vi "gripper.vi"() -> ()   [LabVIEW 2017]
uses:
  Program Files (x86)/National Instruments/LabVIEW 2017/examples/Instrument IO/Serial/support/Serial - Settings.ctl
  <vilib>/Instr/_visa.llb/VISA Configure Serial Port (Instr).vi
panel:
  in  "열림":bool
  in  "닫힘":bool
  out "입력":string="*IDN?\n"
  in  "정지":bool
  out "Response":string
  out "bytes read":u32
  out "check":bool
  in  "Serial Settings":T1={"baud rate"=9600, "data bits"=8, "parity"=enum."None", "stop bits"=10, "flow control"=0} {"flow control" items=["None"=0, "XON/XOFF"=1, "RTS/CTS"=2, "DTR/DSR"=4]; "stop bits" items=["1.0"=10, "1.5"=15, "2.0"=20]; "data bits" min=5 max=8 step=1; "baud rate" items=["75"=75, "110"=110, "134"=134, "150"=150, "300"=300, "600"=600, "1200"=1200, "1800"=1800, "2400"=2400, "4800"=4800, "7200"=7200, "9600"=9600, "14400"=14400, "19200"=19200, "28800"=28800, "38400"=38400, "56000"=56000, "57600"=57600, "115200"=115200, "128000"=128000, "230400"=230400]}
  in  "delay before read (ms)":u32=500
  in  "VISA resource name":refnum<visa-resource-name>="COM1"
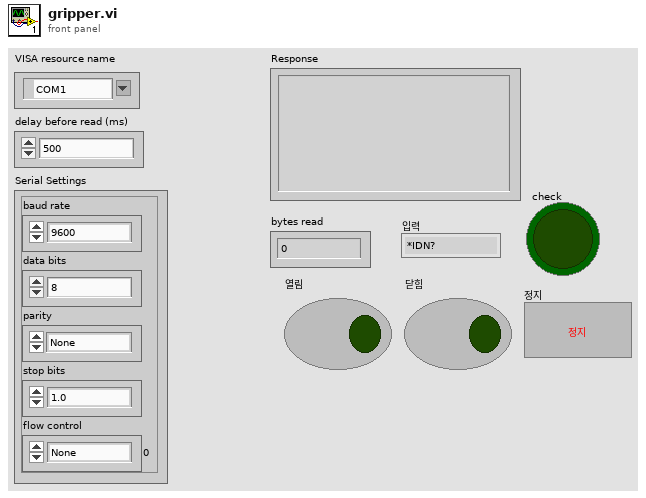
[diagram p1: front panel]
types:
  T1 = typedef "Serial - Settings.ctl" = cluster{"baud rate":u32, "data bits":u16, "parity":enum16{"None", "Odd", "Even", "Mark", "Space"}, "stop bits":u16, "flow control":u16}
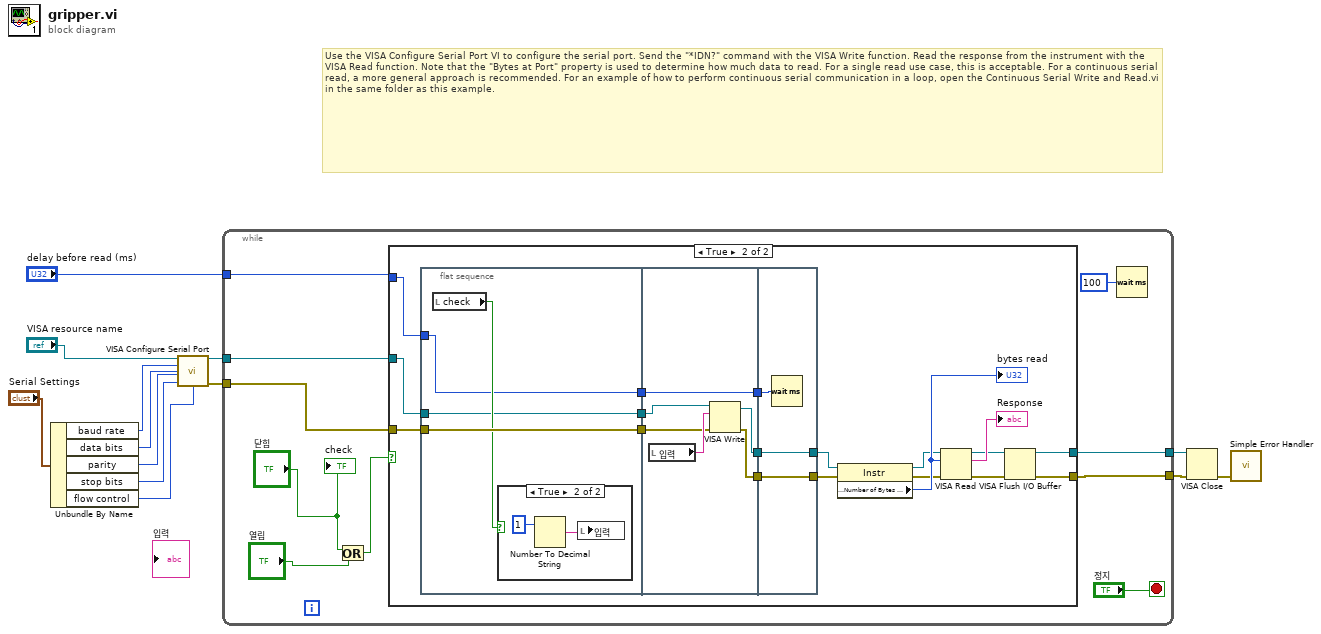
[diagram p0: block diagram]
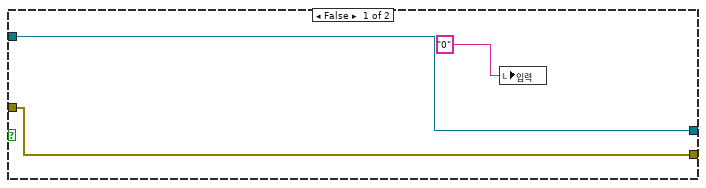
[diagram p2: hidden frame]
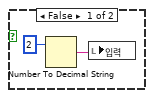
[diagram p3: hidden frame]
diagram:
  # "Use the VISA Configure Serial Port VI to configure the serial port. Send the \"*IDN?\" command with the VISA Write function. Read the response from the instrument with the VISA Read function. Note that the \"Bytes at Port\" property is used to determine how much data to read. For a single read use case, this is acceptable. For a continuous serial read, a more general approach is recommended. For an example of how to perform continuous serial communication in a loop, open the Continuous Serial Write and Read.vi in the same folder as this example."
  n1 = Unbundle By Name("Serial Settings") -> ("baud rate"=w10:u32, "data bits"=w9:u16, "parity"=w8:enum16{"None", "Odd", "Even", "Mark", "Space"}, "stop bits"=w7:u16, "flow control"=w6:u16)
  n2 = call-poly "VISA Configure Serial Port"("VISA resource name"="VISA resource name", "baud rate (9600)"=w10, "data bits (8)"=w9, "parity (0:none)"=w8, "stop bits (10: 1 bit)"=w7, "flow control (0:none)"=w6) -> ("VISA resource name out"=w5:refnum<visa-resource-name>, "error out"=w4:errorcluster)  [unwired: 3 in, 5 out]
  n3 = while {
    tunnel: "delay before read (ms)" -> [w20]
    tunnel: w5 -> [w18]
    tunnel: w4 -> [w19]
    tunnel: [w17] -> w3
    tunnel: [w16] -> w2
    stop <- "정지" stop-if-true
    n4 = Or(x="닫힘", y="열림") -> (x .or. y?=w21:bool)
    n5 = case shown="True" w21 {
      tunnel: w20 -> [_ w35]
      tunnel: [w25 w28] -> w17
      tunnel: w19 -> [w25 w37]
      tunnel: w18 -> [w24 w31]
      tunnel: [w24 w27] -> w16
      frame False {
        n6 = local write "입력"("0") -> ()
      }
      frame True {
        n7 = flat-sequence {
          tunnel: w37 -> [w49]
          tunnel: [w49] -> w36
          tunnel: w35 -> [w47]
          tunnel: [w47] -> w33
          tunnel: [w46] -> w32
          tunnel: w31 -> [w46]
          tunnel: [w57] -> w39
          tunnel: [w56] -> w38
          tunnel: w36 -> [w58]
          tunnel: [w55] -> w34
          tunnel: w33 -> [w55]
          tunnel: w32 -> [w54]
          tunnel: [w62] -> w40
          tunnel: [w61] -> w41
          tunnel: w39 -> [w62]
          tunnel: w38 -> [w61]
          tunnel: w34 -> [w60]
          frame #0 {
            n8 = local read "check"() -> (w48:bool)
            n9 = case shown="True" w48 {
              frame False {
                n10 = Number To Decimal String(number=2 ("숫자")) -> (decimal integer string=w51:string)  [unwired: 1 in]
                n11 = local write "입력"(w51) -> ()
              }
              frame True {
                n12 = Number To Decimal String(number=1 ("숫자")) -> (decimal integer string=w53:string)  [unwired: 1 in]
                n13 = local write "입력"(w53) -> ()
              }
            }
          }
          frame #1 {
            n14 = local read "입력"() -> (w59:string)
            n15 = VISA Write(VISA resource name=w54, write buffer=w59, error in (no error)=w58) -> (VISA resource name out=w56:refnum<visa-resource-name>, error out=w57:errorcluster)  [unwired: 1 out]
          }
          frame #2 {
            n16 = Wait (ms)(milliseconds to wait=w60) -> ()  [unwired: 1 out]
          }
        }
        n17 = property class="Instr"(reference=w41, error in=w40) -> (reference out=w42:refnum<visa-resource-name>, error out=w43:errorcluster, "Serial Settings:Number of Bytes at Serial Port"=w45:u32)
        "bytes read" <- w45
        n18 = VISA Read(VISA resource name=w42, byte count=w45, error in (no error)=w43) -> (VISA resource name out=w30:refnum<visa-resource-name>, read buffer=→"Response":string, error out=w29:errorcluster)  [unwired: 1 out]
        n19 = VISA Flush I/O Buffer(VISA resource name=w30, error in (no error)=w29) -> (VISA resource name out=w27:refnum<visa-resource-name>, error out=w28:errorcluster)  [unwired: 1 in]
      }
    }
    n20 = Wait (ms)(milliseconds to wait=u32 100 ("대기 시간 (ms)")) -> ()  [unwired: 1 out]
    "check" <- "닫힘"
  }
  n21 = VISA Close(VISA resource name=w2, error in (no error)=w3) -> (error out=w1:errorcluster)
  n22 = call <vilib>:"Simple Error Handler.vi"("error in (no error)"=w1) -> ()  [unwired: 1 in, 8 out]
